vi "UI Ref FG.vi"(10 "Slide In":refnum<vi>, 11 "Iteration In":refnum<vi>) -> (0 "error out":errorcluster, 2 "Slide":refnum<vi>, 3 "Iteration":refnum<vi>)   [LabVIEW 2020]
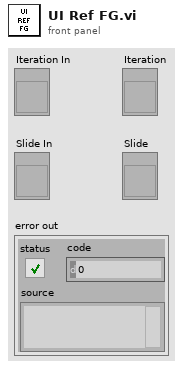
[diagram p1: front panel]
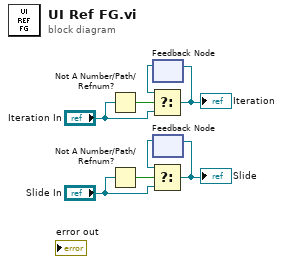
[diagram p0: block diagram]
diagram:
  n1 = Not A Number/Path/Refnum?(number/path/refnum="Iteration In") -> (NaN/Path/Refnum?=w8:bool)
  n2 = Not A Number/Path/Refnum?(number/path/refnum="Slide In") -> (NaN/Path/Refnum?=w2:bool)
  n3 = feedback #1() -> (w5:refnum<vi>)  [unwired: 1 in]
  n4 = Select(t=w5, s=w8, f="Iteration In") -> (s? t:f=w6:refnum<vi>)
  "Iteration" <- w6
  n5 = feedback-in #1(w6) -> ()
  n6 = feedback #2() -> (w4:refnum<vi>)  [unwired: 1 in]
  n7 = Select(t=w4, s=w2, f="Slide In") -> (s? t:f=w3:refnum<vi>)
  "Slide" <- w3
  n8 = feedback-in #2(w3) -> ()
